vi "Keithley2100.ProcEvents.vi"(0 "i ref in":refnum<vi>, 5 "error in (no error)":errorcluster) -> (14 "i ref out":refnum<vi>, 19 "error out":errorcluster)   [LabVIEW 2014, in "Keithley2100.lvlib"]
doc: "This method is used to define the events the object will listen to. Add your own events here."
uses:
  Keithley2100.lvlib
  CS_Core/BaseProcess/BaseProcess.event definition.ctl
  CS_Core/CAEObj/CAEObj.event definition.ctl
  CS_Core/BaseProcess/BaseProcess.descriptor string definition.ctl
  CS_Core/BaseProcess/BaseProcess.lvlib
  CS_Core/CAEObj/CAEObj.lvlib
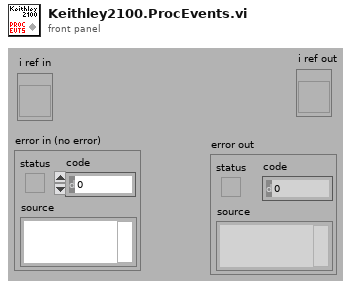
[diagram p1: front panel]
types:
  T1 = typedef "BaseProcess.lvlib/BaseProcess.event definition.ctl" = cluster{"CAEEvtDef":T2, "Data Descriptor":T3}
  T2 = typedef "CAEObj.lvlib/CAEObj.event definition.ctl" = cluster{"URL":string, "enable":bool, "ignoreResID":bool}
  T3 = typedef "BaseProcess.lvlib/BaseProcess.descriptor string definition.ctl" = string
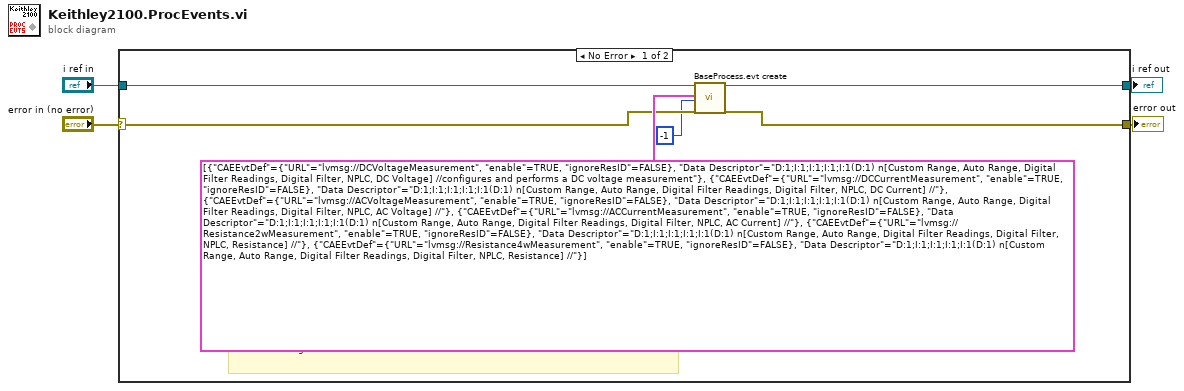
[diagram p0: block diagram]
diagram:
  n1 = case shown="No Error" "error in (no error)" {
    selector: "error in (no error)" -> [w6 w11]
    tunnel: "i ref in" -> [w10 w12]
    tunnel: [w9 w12] -> w3
    tunnel: [w8 w11] -> w2
    frame No Error {
      # "Example add is just an example for your function\nThe format is the following:\n1) event selector (that is the selector that will be used later when an event has arrived)\n2) event URL that specifies not only the name of the URL but also the protocol used.\n3) boolean flag to enable/disable the event."
      n2 = call "BaseProcess.evt create.vi"("i ref in"=w10, "newEvents"=T1[] [{"CAEEvtDef"={"URL"="lvmsg://DCVoltageMeasurement", "enable"=TRUE, "ignoreResID"=FALSE}, "Data Descriptor"="D:1;I:1;I:1;I:1;I:1(D:1) n[Custom Range, Auto Range, Digital Filter Readings, Digital Filter, NPLC, DC Voltage] //configures and performs a DC voltage measurement"}, {"CAEEvtDef"={"URL"="lvmsg://DCCurrentMeasurement", "enable"=TRUE, "ignoreResID"=FALSE}, "Data Descriptor"="D:1;I:1;I:1;I:1;I:1(D:1) n[Custom Range, Auto Range, Digital Filter Readings, Digital Filter, NPLC, DC Current] //"}, {"CAEEvtDef"={"URL"="lvmsg://ACVoltageMeasurement", "enable"=TRUE, "ignoreResID"=FALSE}, "Data Descriptor"="D:1;I:1;I:1;I:1;I:1(D:1) n[Custom Range, Auto Range, Digital Filter Readings, Digital Filter, NPLC, AC Voltage] //"}, {"CAEEvtDef"={"URL"="lvmsg://ACCurrentMeasurement", "enable"=TRUE, "ignoreResID"=FALSE}, "Data Descriptor"="D:1;I:1;I:1;I:1;I:1(D:1) n[Custom Range, Auto Range, Digital Filter Readings, Digital Filter, NPLC, AC Current] //"}, {"CAEEvtDef"={"URL"="lvmsg://Resistance2wMeasurement", "enable"=TRUE, "ignoreResID"=FALSE}, "Data Descriptor"="D:1;I:1;I:1;I:1;I:1(D:1) n[Custom Range, Auto Range, Digital Filter Readings, Digital Filter, NPLC, Resistance] //"}, {"CAEEvtDef"={"URL"="lvmsg://Resistance4wMeasurement", "enable"=TRUE, "ignoreResID"=FALSE}, "Data Descriptor"="D:1;I:1;I:1;I:1;I:1(D:1) n[Custom Range, Auto Range, Digital Filter Readings, Digital Filter, NPLC, Resistance] //"}] ("new events"), "ms timeout (10000)"=-1, "error in (no error)"=w6) -> ("i ref out"=w9:refnum<vi>, "error out"=w8:errorcluster)  [unwired: 12 in, 2 out]
    }
    frame Error {
    }
  }
  "i ref out" <- w3
  "error out" <- w2
